vi "hpcnc move Y.vi"(0 "VISA Refnum in":refnum<visa-resource-name>, 1 "Y":dbl, 4 "Speed":i32=100, 5 "error in":errorcluster) -> (14 "VISA Refnum out":refnum<visa-resource-name>, 19 "error out":errorcluster)   [LabVIEW 2014]
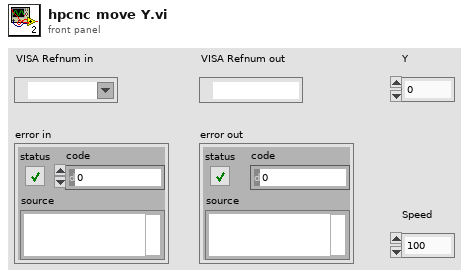
[diagram p1: front panel]
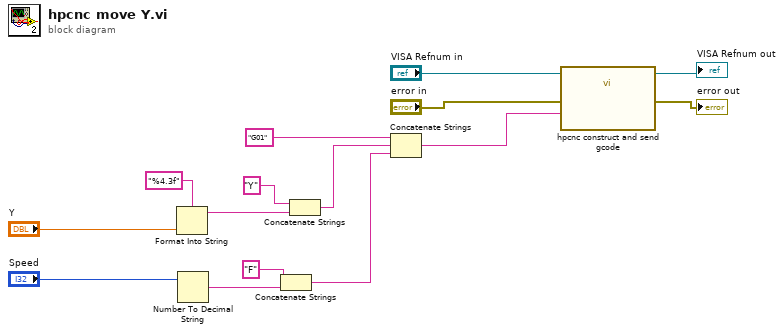
[diagram p0: block diagram]
diagram:
  n1 = Format Into String(format string="%4.3f", "Y") -> (resulting string=w8:string)  [unwired: 2 in, 1 out]
  n2 = Number To Decimal String(number="Speed") -> (decimal integer string=w5:string)  [unwired: 1 in]
  n3 = Concatenate Strings("F" ("string"), w5) -> (w4:string)
  n4 = Concatenate Strings("Y" ("string"), w8) -> (w7:string)
  n5 = Concatenate Strings("G01" ("string"), w7, w4) -> (w1:string)
  n6 = call "hpcnc construct and send gcode.vi"("error in (no error)"="error in", "GCode"=w1, "VISA Refnum in"="VISA Refnum in") -> ("error out"=→"error out":errorcluster, "VISA Refnum out"=→"VISA Refnum out":refnum<visa-resource-name>)  [unwired: 7 in]
